vi "Image Transfer RT to FPGA (SubVI).vi"(7 "error in (no error)":errorcluster, 8 "Image to Transfer In":T2, 9 "Image Size In":T1, 10 "Custom FPGA Reference In":refnum<k20>) -> (0 "error out":errorcluster, 1 "Empty Elements Remaining":u32, 2 "Image Size Out":T1, 3 "Custom FPGA Reference Out":refnum<k20>)   [LabVIEW 2017, in "SoC IP Library.lvlib"]
uses:
  SoC IP Library.lvlib
  Controls/Image Size.ctl
  <vilib>/vision/Image Controls.llb/IMAQ Image.ctl
  <vilib>/Utility/error.llb/Error Cluster From Error Code.vi
  <vilib>/rvi/errors/niLvFpgaAdjustHostInterfaceError.vi
  <vilib>/rvi/interface/nirviMethod/nirviMethod.xnode
  <vilib>/vision/NI_Vision_Development_Module.lvlib
  <vilib>/FPGAPlugInAG/Dynamic/niLvFpga_WriteFifo_Dynamic.vi
  <vilib>/rvi/errors/niLvFpgaMergeErrorWithErrorCode.vi
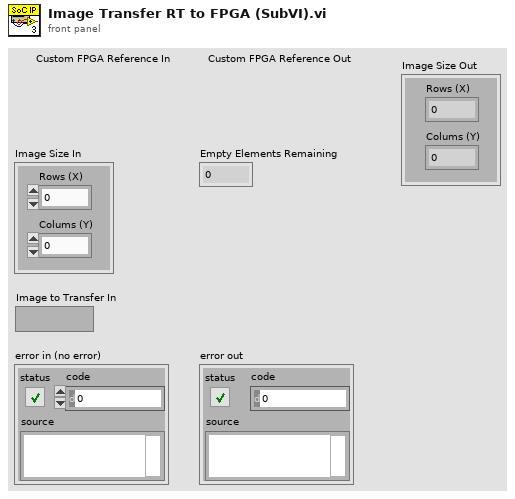
[diagram p1: front panel]
types:
  T1 = typedef "SoC IP Library.lvlib/Image Size.ctl" = cluster{"Rows (X)":u16, "Colums (Y)":u16}
  T2 = typedef "IMAQ Image.ctl" = refnum<image>
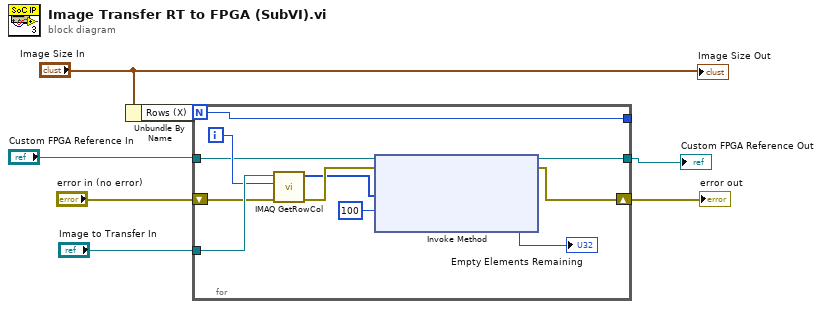
[diagram p0: block diagram]
diagram:
  n1 = Unbundle By Name("Image Size In") -> ("Rows (X)"=w6:u16)
  n2 = for {
    N: w6 -> [w12]
    shift-right: [w11] -> w4
    shift-left: "error in (no error)" -> [w15]
    tunnel: "Image to Transfer In" -> [w17]
    tunnel: [w18] -> w2
    tunnel: [w12] -> _
    tunnel: "Custom FPGA Reference In" -> [w10]
    i -> [w16]
    n3 = call "IMAQ GetRowCol"("Image"=w17, "Number"=w16, "error in (no error)"=w15) -> ("Pixels (U8)"=w9:u8[], "error out"=w14:errorcluster)  [unwired: 3 in, 3 out]
    n4 = xnode "Invoke Method"("FPGA VI Reference In"=w10, "error in"=w14, "Data"=w9, "Timeout (ms)"=100) -> ("FPGA VI Reference Out"=w18:refnum<k20>, "error out"=w11:errorcluster, "Empty Elements Remaining"=→"Empty Elements Remaining":u32)
  }
  "error out" <- w4
  "Custom FPGA Reference Out" <- w2
  "Image Size Out" <- "Image Size In"
